vi "8164B CloseLANConnection.vi"(8 "error in":errorcluster, 11 "KeySight 8164B control":T1) -> (0 "error out":errorcluster)   [LabVIEW 2018, in "KeySight 8164B LAN InstrLib.lvlib"]
uses:
  KeySight 8164B LAN InstrLib.lvlib
  typedefs/KeySight 8164B control.ctl
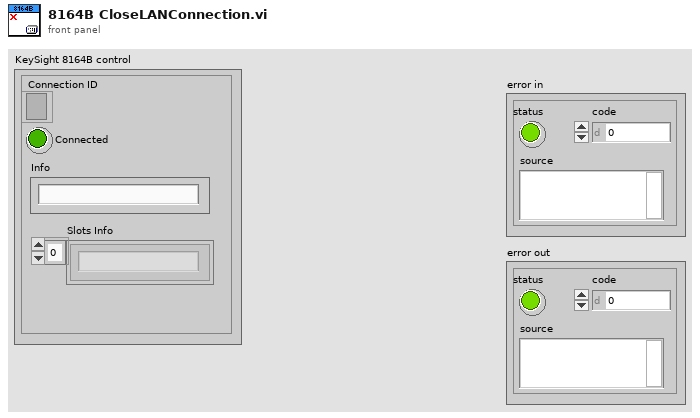
[diagram p1: front panel]
types:
  T1 = typedef "KeySight 8164B LAN InstrLib.lvlib/KeySight 8164B control.ctl" = cluster{"Connection ID":refnum<k5>, "Connected":bool, "Info":string, "Slots Info":string[]}
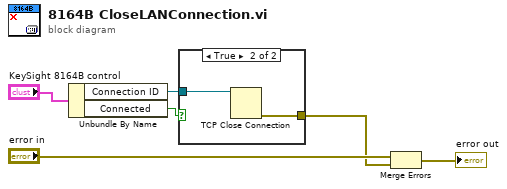
[diagram p0: block diagram]
diagram:
  n1 = Unbundle By Name("KeySight 8164B control") -> ("Connection ID"=w4:refnum<k5>, "Connected"=w5:bool)
  n2 = case shown="True" w5 {
    tunnel: w4 -> [_ w8]
    tunnel: [_ w7] -> w2
    frame False {
    }
    frame True {
      n3 = TCP Close Connection(connection ID=w8) -> (error out=w7:errorcluster)  [unwired: 2 in, 1 out]
    }
  }
  n4 = Merge Errors("error in", w2) -> (→"error out":errorcluster)
